vi "enqueData.vi"(8 "error in (no error)":errorcluster, 9 "Queue Reference":refnum<queue>, 10 "Descriptor":string, 11 "Value IN":dbl) -> (0 "error out":errorcluster)   [LabVIEW 2016]
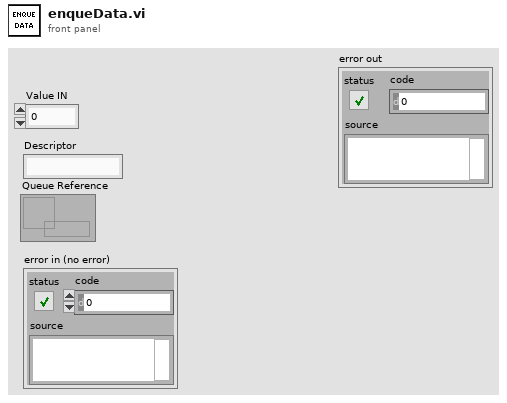
[diagram p1: front panel]
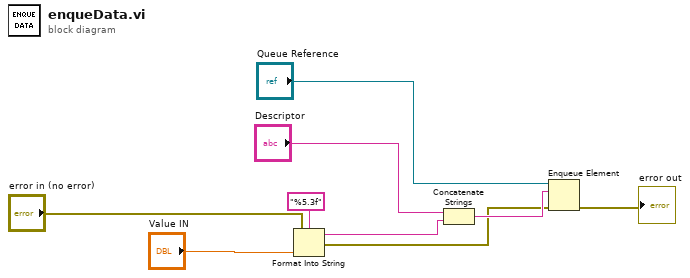
[diagram p0: block diagram]
diagram:
  n1 = Format Into String(format string="%5.3f", error in="error in (no error)", "Value IN") -> (resulting string=w6:string, error out=w2:errorcluster)  [unwired: 1 in]
  n2 = Concatenate Strings("Descriptor", w6) -> (w7:string)
  n3 = Enqueue Element(queue="Queue Reference", element=w7, error in (no error)=w2) -> (error out=→"error out":errorcluster)  [unwired: 1 in, 2 out]
